vi "MSScript_SubVI_GetShowArray.vi"(11 "VarString in":string) -> (1 "ArrayVariable out":ext[](array[numeric]), 2 "Index":i32[](array[numeric]), 3 "ShowName":string, 4 "Is a variable ?":bool, 6 "Value Error?":bool)   [LabVIEW 2018, in "MSScript.lvclass"]
uses:
  MSScript/MSScript.lvclass
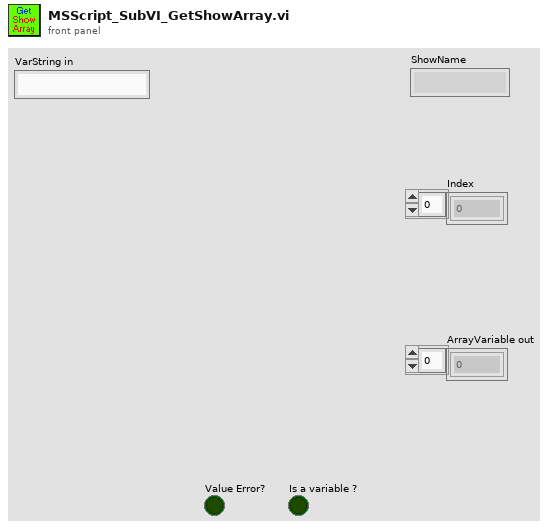
[diagram p1: front panel]
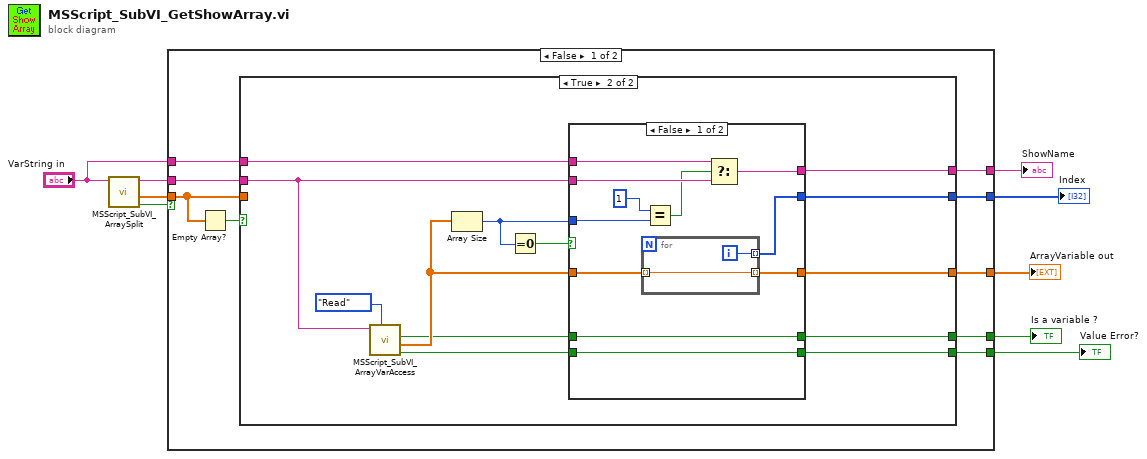
[diagram p0: block diagram]
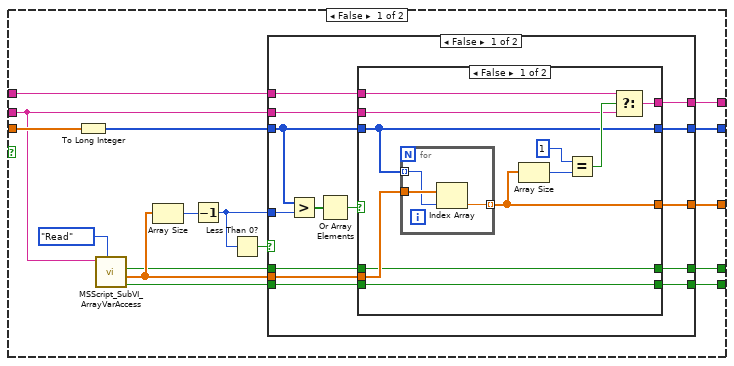
[diagram p2: hidden frame]
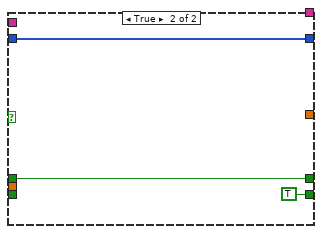
[diagram p3: hidden frame]
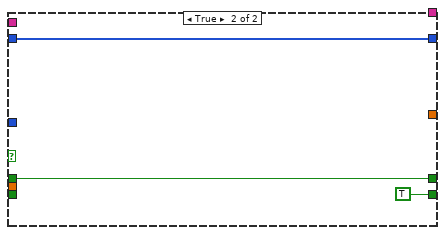
[diagram p4: hidden frame]
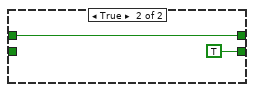
[diagram p5: hidden frame]
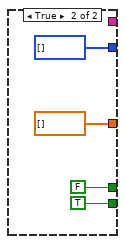
[diagram p6: hidden frame]
diagram:
  n1 = call "MSScript_SubVI_ArraySplit.vi"("VarString in"="VarString in") -> ("Value Error?"=w9:bool, "ArrayVariable out"=w7:ext[], "@name"=w8:string)  [unwired: 7 in, 1 out]
  n2 = case shown="False" w9 {
    tunnel: w8 -> [w17 _]
    tunnel: w7 -> [w14 _]
    tunnel: [w16 FALSE ("Is a variable ?")] -> w5
    tunnel: [w15 TRUE ("Value Error?")] -> w4
    tunnel: [w13 i32[] []] -> w6
    tunnel: [w12 ext[] [] ("ArrayVariable out")] -> w1
    tunnel: "VarString in" -> [w11 _]
    tunnel: [w10 _] -> w2
    frame False {
      n3 = Empty Array?(array=w14) -> (empty?=w18:bool)
      n4 = case shown="True" w18 {
        tunnel: w17 -> [w29 w79]
        tunnel: [w24 w72] -> w16
        tunnel: [w22 w70] -> w15
        tunnel: w14 -> [w33 _]
        tunnel: [w20 w75] -> w13
        tunnel: [w31 w76] -> w12
        tunnel: w11 -> [w30 w80]
        tunnel: [w28 w78] -> w10
        frame False {
          n5 = To Long Integer(number=w33) -> (32bit integer=w32:i32[])
          n6 = call "MSScript_SubVI_ArrayVarAccess.vi"("Function (Read)"=enum16{"Init", "Write", "Read"}."Read", "VarName"=w29) -> ("Value Error?"=w23:bool, "ArrayVariable out"=w27:ext[], "Is a variable ?"=w25:bool)  [unwired: 5 in]
          n7 = Array Size(array=w27) -> (size(s)=w26:i32)
          n8 = Decrement(x=w26) -> (x-1=w19:i32)
          n9 = Less Than 0?(x=w19) -> (x < 0?=w21:bool)
          n10 = case shown="False" w21 {
            tunnel: w32 -> [w43 w66]
            tunnel: [w48 _] -> w31
            tunnel: w30 -> [w47 _]
            tunnel: w29 -> [w46 _]
            tunnel: [w45 _] -> w28
            tunnel: w27 -> [w44 _]
            tunnel: w25 -> [w40 w68]
            tunnel: [w39 w68] -> w24
            tunnel: w23 -> [w38 _]
            tunnel: [w37 TRUE ("Value Error?")] -> w22
            tunnel: [w35 w66] -> w20
            tunnel: w19 -> [w42 _]
            frame False {
              n11 = Greater?(x=w43, y=w42) -> (0:w41:bool[])
              n12 = Or Array Elements(Boolean array=w41) -> (logical OR=w36:bool)
              n13 = case shown="False" w36 {
                tunnel: [w59 _] -> w48
                tunnel: w47 -> [w55 _]
                tunnel: w46 -> [w54 _]
                tunnel: [w53 _] -> w45
                tunnel: w44 -> [w52 _]
                tunnel: w43 -> [w49 w65]
                tunnel: w40 -> [w51 w64]
                tunnel: [w51 w64] -> w39
                tunnel: w38 -> [w50 _]
                tunnel: [w50 TRUE ("Value Error?")] -> w37
                tunnel: [w49 w65] -> w35
                frame False {
                  n14 = for {
                    tunnel: w49 -> [w61] mode=indexing
                    tunnel: w52 -> [w62]
                    tunnel: [w60] -> w59 mode=indexing
                    n15 = Index Array(array=w62, index=w61) -> (element=w60:ext)
                  }
                  n16 = Array Size(array=w59) -> (size(s)=w58:i32)
                  n17 = Equal?(x=1, y=w58) -> (x = y?=w56:bool)
                  n18 = Select(t=w55, s=w56, f=w54) -> (s? t:f=w53:string)
                }
                frame True {
                }
              }
            }
            frame True {
            }
          }
        }
        frame True {
          n19 = call "MSScript_SubVI_ArrayVarAccess.vi"("Function (Read)"=enum16{"Init", "Write", "Read"}."Read", "VarName"=w79) -> ("Value Error?"=w71:bool, "ArrayVariable out"=w77:ext[], "Is a variable ?"=w73:bool)  [unwired: 5 in]
          n20 = Array Size(array=w77) -> (size(s)=w74:i32)
          n21 = Equal To 0?(x=w74) -> (x = 0?=w69:bool)
          n22 = case shown="False" w69 {
            tunnel: w80 -> [w91 _]
            tunnel: w79 -> [w90 _]
            tunnel: [w88 _] -> w78
            tunnel: w77 -> [w87 _]
            tunnel: [w86 _] -> w76
            tunnel: [w85 _] -> w75
            tunnel: w74 -> [w84 _]
            tunnel: w73 -> [w83 w96]
            tunnel: [w83 w96] -> w72
            tunnel: w71 -> [w82 _]
            tunnel: [w82 TRUE ("Value Error?")] -> w70
            frame False {
              n23 = for {
                tunnel: w87 -> [w94] mode=indexing
                tunnel: [w94] -> w86 mode=indexing
                tunnel: [w93] -> w85 mode=indexing
                i -> [w93]
              }
              n24 = Equal?(x=1, y=w84) -> (x = y?=w89:bool)
              n25 = Select(t=w91, s=w89, f=w90) -> (s? t:f=w88:string)
            }
            frame True {
            }
          }
        }
      }
    }
    frame True {
    }
  }
  "Index" <- w6
  "Is a variable ?" <- w5
  "Value Error?" <- w4
  "ShowName" <- w2
  "ArrayVariable out" <- w1
